vi "z shm client storage clone.vi"(8 "error in (no error)":errorcluster, 10 "from":cluster{}, 11 "this_":cluster{}) -> (0 "error out":errorcluster, 3 "this_ out":cluster{})   [LabVIEW 2021, in "zenohc.lvlib"]
doc: "void z_shm_client_storage_clone(struct z_owned_shm_client_storage_t *this_,\n const struct z_loaned_shm_client_storage_t *from);"
uses:
  zenohc.lvlib
  zenohc.dll
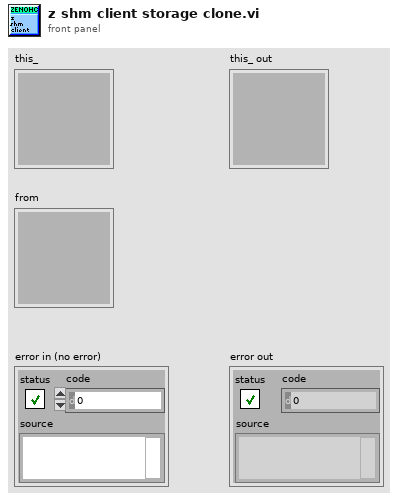
[diagram p1: front panel]
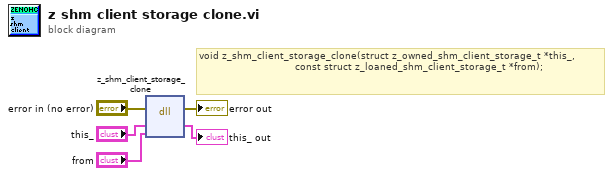
[diagram p0: block diagram]
diagram:
  # "void z_shm_client_storage_clone(struct z_owned_shm_client_storage_t *this_,\n                                const struct z_loaned_shm_client_storage_t *from);"
  n1 = dll-call lib="D:/dev/zenoh_labview/zenohc/zenohc.*" fn="z_shm_client_storage_clone"(error in="error in (no error)", "this_"="this_", "from"="from") -> (error out=→"error out":errorcluster, "this_"=→"this_ out":cluster{})  [unwired: 4 in, 1 out]
